vi "Untitled 8 (SubVI) 1.vi"(6 "Array 2":dbl[](array[numeric]), 7 "Array 3":dbl[](array[numeric]), 9 "Array":dbl[](array[numeric]), 10 "Array 6":dbl[](array[numeric]), 11 "Array 5":dbl[](array[numeric])) -> (1 "ZICHT  functie":cluster{"Y":dbl[], "Y":dbl[]}[](graph), 2 "free gas model":cluster{"Y":dbl[], "Y":dbl[]}[](graph), 3 "core electrons":cluster{"Y":dbl[], "Y":dbl[]}[](graph))   [LabVIEW 2013]
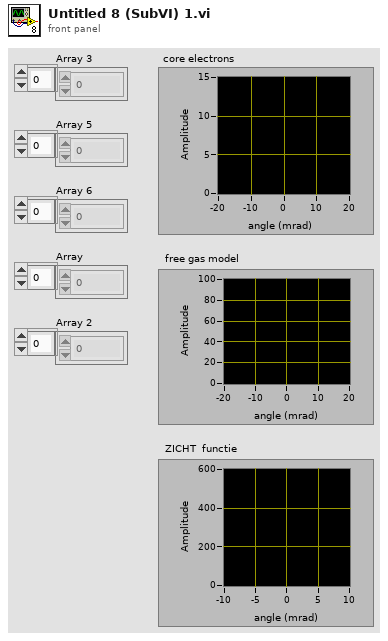
[diagram p1: front panel]
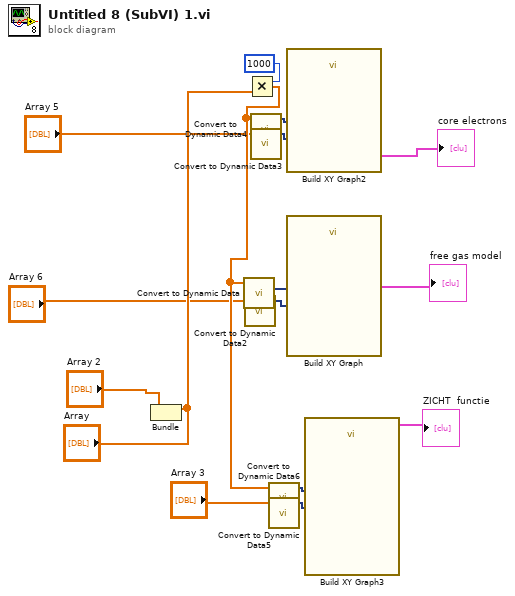
[diagram p0: block diagram]
diagram:
  n1 = Bundle("Array"="Array", "Array 2"="Array 2") -> ()  [unwired: 1 in, 1 out]
  n2 = call "Convert to Dynamic Data2"("Array"="Array 6") -> ("Dynamic Data Type"=w2:dynamicdata)  [unwired: 3 in]
  n3 = Multiply(x=1000, y="Array") -> (x*y=w15:dbl[])
  n4 = call "Convert to Dynamic Data"("Array"=w15) -> ("Dynamic Data Type"=w3:dynamicdata)  [unwired: 3 in]
  n5 = call "Convert to Dynamic Data4"("Array"=w15) -> ("Dynamic Data Type"=w8:dynamicdata)  [unwired: 3 in]
  n6 = call "Convert to Dynamic Data3"("Array"="Array 5") -> ("Dynamic Data Type"=w7:dynamicdata)  [unwired: 3 in]
  n7 = call "Convert to Dynamic Data6"("Array"=w15) -> ("Dynamic Data Type"=w11:dynamicdata)  [unwired: 3 in]
  n8 = call "Convert to Dynamic Data5"("Array"="Array 3") -> ("Dynamic Data Type"=w10:dynamicdata)  [unwired: 3 in]
  n9 = call "Build XY Graph2"("Y Input"=w7, "X Input"=w8) -> ("XY Graph"=→"core electrons":cluster{"Y":dbl[], "Y":dbl[]}[])  [unwired: 8 in, 1 out]
  n10 = call "Build XY Graph"("Y Input"=w2, "X Input"=w3) -> ("XY Graph"=→"free gas model":cluster{"Y":dbl[], "Y":dbl[]}[])  [unwired: 8 in, 1 out]
  n11 = call "Build XY Graph3"("Y Input"=w10, "X Input"=w11) -> ("XY Graph"=→"ZICHT  functie":cluster{"Y":dbl[], "Y":dbl[]}[])  [unwired: 8 in, 1 out]
